vi "Ruleredge.vi"(7 "error in":errorcluster) -> (20 "Edge Information (Edge Detector 1)":T2[](array[typedef]) {"Distance (Real-World)" format="%.2f"; "Location (Real-World)"."Y" format="%.2g"; "Location (Real-World)"."X" format="%.2f"; "Noise" format="%.2f"; "Location (Pixel)"."Y" format="%.2g"; "Location (Pixel)"."X" format="%.2f"; "Strength" format="%.2f"; "Distance (Pixel)" format="%.2f"}, 21 "Caliper Results (Ruler Width)":sgl[][](array[numeric]) format="%.2f", 22 "Calibrated Results (Ruler Width)":sgl[][](array[numeric]) format="%.2f", 27 "error out":errorcluster)   [LabVIEW 2015]
uses:
  <vilib>/vision/Measure.llb/Edge New.ctl
  <vilib>/vision/NI_Vision_Development_Module.lvlib
panel:
  out "Image Out":T1(plugin-control)
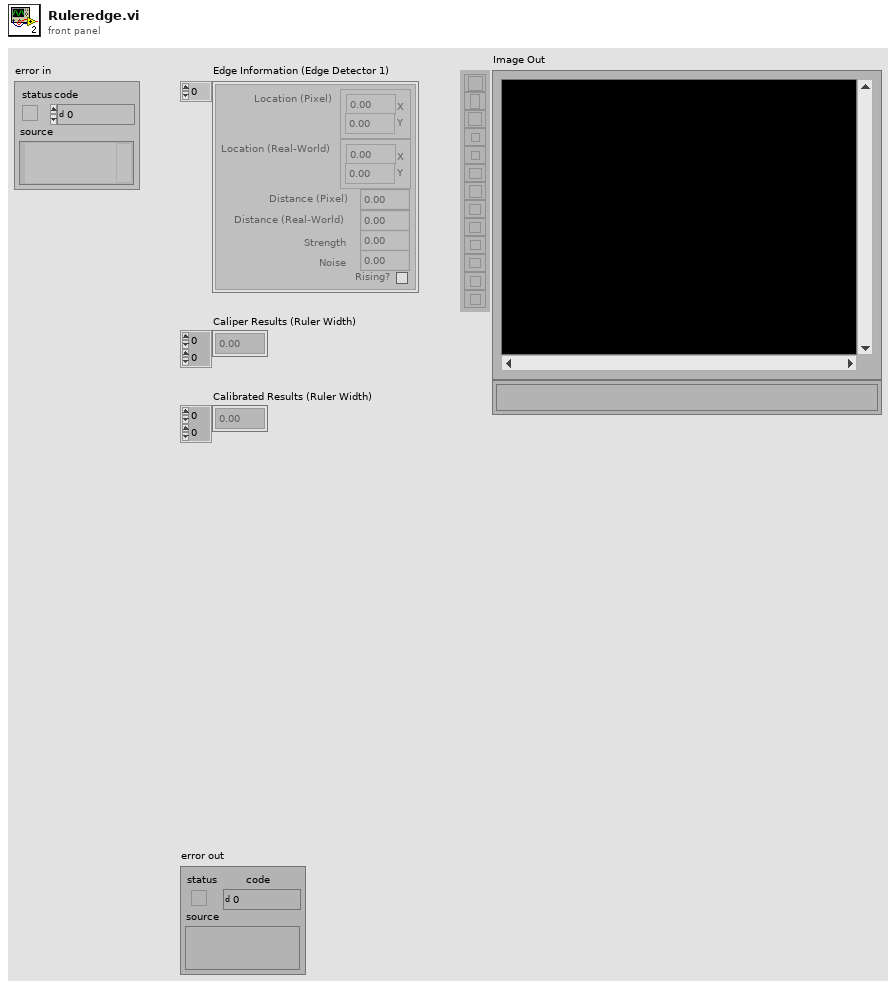
[diagram p1: front panel]
types:
  T1 = typedef "IMAQ Image.ctl" = refnum<image>
  T2 = typedef "Edge New.ctl" = cluster{"Location (Pixel)":cluster{"X":sgl, "Y":sgl}, "Location (Real-World)":cluster{"X":sgl, "Y":sgl}, "Distance (Pixel)":dbl, "Distance (Real-World)":dbl, "Strength":dbl, "Noise":dbl, "Rising?":bool}
  T3 = cluster{"Feature":u32, "Points IDs":cluster{"GUID":string, "Index":i32}[]}[]
  T4 = cluster{"Edge Polarity":u32, "Kernel Size":u32, "Width":u32, "Minimum Edge Strength":sgl, "Interpolation Type":enum32{"Zero Order", "Bilinear", "Quadratic", "Cubic", "Bilinear Fixed"}, "Data Processing Method":enum32{"Average", "Median"}}
  T5 = enum16{"Get First Edge", "Get First + Last Edge", "Get All Edges", "Get Best Edge"}
  T6 = cluster{"Global Rectangle":i32[], "Contours":cluster{"ID":enum32{"External", "Internal"}, "Type":u32, "Coordinates":i32[]}[]}
  T7 = typedef "Image Type" = u32
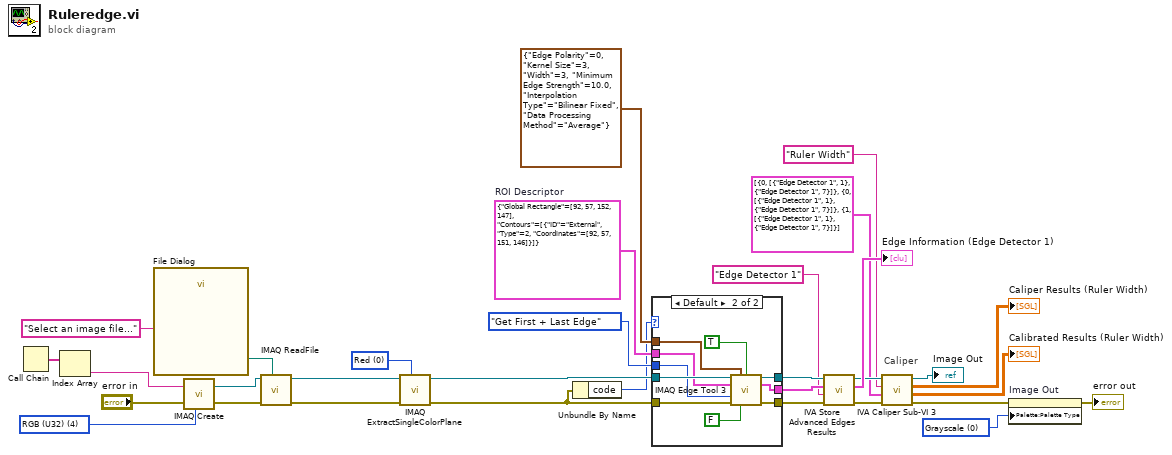
[diagram p0: block diagram]
diagram:
  w1 = u32 0 items=["Grayscale", "Binary", "Gradient", "Rainbow", "Temperature", "User Defined", "Binary 16 Bit", "Gradient 16 Bit", "Rainbow 16 Bit", "Temperature 16 Bit", "User Defined 16 Bit"] ("Palette Type")
  w13 = T6 {"Global Rectangle"=[92, 57, 152, 147], "Contours"=[{"ID"=enum."External", "Type"=2, "Coordinates"=[92, 57, 151, 146]}]}  # ROI Descriptor
  w24 = 0 items=["Red", "Green", "Blue", "Hue", "Saturation", "Luminance", "Value", "Intensity"] ("Color Plane")
  w25 = T7 4 items=["Grayscale (U8)", "Grayscale (I16)", "Grayscale (SGL)", "Complex (CSG)", "RGB (U32)", "HSL (U32)", "RGB (U64)", "Grayscale (U16)"] ("Image Type")
  # "Caliper"
  n1 = Call Chain() -> (call chain=w29:string[])
  n2 = Index Array(array=w29) -> (element=w28:string)  [unwired: 1 in]
  n3 = call "File Dialog"("prompt"="Select an image file...") -> ("selected path"=w26:path)  [unwired: 6 in, 8 out]
  n4 = call "IMAQ Create"("Image Name"=w28, "Image Type"=w25, "error in (no error)"="error in") -> ("New Image"=w32:T1, "error out"=w31:errorcluster)  [unwired: 1 in, 1 out]
  n5 = call "IMAQ ReadFile"("File Path"=w26, "error in (no error)"=w31, "Image"=w32) -> ("error out"=w22:errorcluster, "Image Out"=w23:T1)  [unwired: 2 in, 5 out]
  n6 = call "IMAQ ExtractSingleColorPlane"("Color Plane"=w24, "error in (no error)"=w22, "Image Src"=w23) -> ("error out"=w12:errorcluster, "Image Dst Out"=w21:T1)  [unwired: 1 in, 6 out]
  n7 = Unbundle By Name(w12) -> ("code"=w11:i32)
  n8 = case shown="Default" w11 {
    tunnel: w12 -> [_ w43]
    tunnel: w21 -> [w33 w42]
    tunnel: T5."Get First + Last Edge" ("Process") -> [_ w41]
    tunnel: T4 {"Edge Polarity"=0, "Kernel Size"=3, "Width"=3, "Minimum Edge Strength"=10.0, "Interpolation Type"=enum."Bilinear Fixed", "Data Processing Method"=enum."Average"} ("Edge Options") -> [_ w40]
    tunnel: [_ w39] -> w18
    tunnel: [w33 w38] -> w17
    tunnel: [_ w37] -> w16
    tunnel: w13 -> [_ w36]
    frame -1074396199, -1074396198 {
    }
    frame Default {
      n9 = call "IMAQ Edge Tool 3"("Image"=w42, "Edge Options"=w40, "Optimized Mode"=TRUE, "ROI Descriptor"=w36, "Process"=w41, "error in (no error)"=w43, "Reverse Direction"=FALSE) -> ("Image (duplicate)"=w38:T1, "Edge Information"=w37:T2[], "error out"=w39:errorcluster)  [unwired: 6 out]
    }
  }
  n10 = call <vilib>:"IVA Store Advanced Edges Results.vi"("error in (no error)"=w18, "Step Name"="Edge Detector 1", "Edge Information"=w16, "Image in"=w17) -> ("error out"=w9:errorcluster, "Edge Information dup"=→"Edge Information (Edge Detector 1)":T2[], "Image dup"=w10:T1)  [unwired: 5 out]
  n11 = call <vilib>:"IVA Caliper Sub-VI 3.vi"("error in"=w9, "Parameters"=T3 [{"Feature"=0, "Points IDs"=[{"GUID"="Edge Detector 1", "Index"=1}, {"GUID"="Edge Detector 1", "Index"=7}]}, {"Feature"=0, "Points IDs"=[{"GUID"="Edge Detector 1", "Index"=1}, {"GUID"="Edge Detector 1", "Index"=7}]}, {"Feature"=1, "Points IDs"=[{"GUID"="Edge Detector 1", "Index"=1}, {"GUID"="Edge Detector 1", "Index"=7}]}], "Step Name"="Ruler Width", "Image In"=w10) -> ("error out"=w4:errorcluster, "Results (Calibrated)"=→"Calibrated Results (Ruler Width)":sgl[][], "Results (Pixels)"=→"Caliper Results (Ruler Width)":sgl[][], "Image Out"=→"Image Out":T1)  [unwired: 1 in, 3 out]
  n12 = property on="Image Out" class="ImageControl"(error in=w4, "Palette:Palette Type"=w1) -> (error out=→"error out":errorcluster)  [unwired: 1 in, 1 out]
